vi "IntuitiveSteering_X.vi"(0 "Input":dbl, 5 "Forward Time":dbl, 7 "Phase Shift":dbl, 9 "Max. Amplitude":dbl) -> (4 "Servo Position":T1)   [LabVIEW 2013]
uses:
  My Computer/Controls/Servo Position.ctl
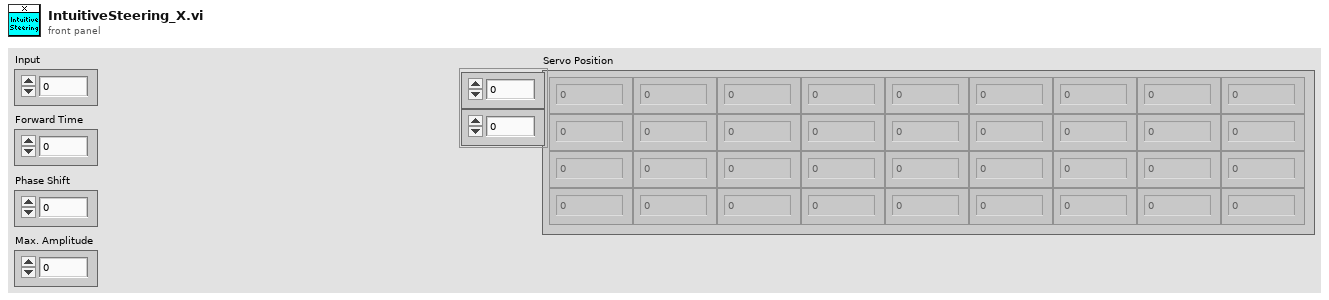
[diagram p1: front panel]
types:
  T1 = typedef "Servo Position.ctl" = dbl[][]
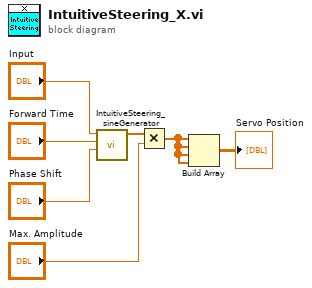
[diagram p0: block diagram]
diagram:
  n1 = call "IntuitiveSteering_sineGenerator.vi"("Phase Shift"="Phase Shift", "Forward Time"="Forward Time", "Input"="Input") -> ("Fin Position"=w4:dbl[])  [unwired: 8 in]
  n2 = Multiply(x=w4, y="Max. Amplitude") -> (x*y=w3:dbl[])
  n3 = Build Array(w3, w3, w3, w3) -> (→"Servo Position":dbl[][])
